vi "Obtain ID from Pool.vi"(8 "error in (no error)":errorcluster, 9 "timeout in ms (0)":i32 format="%d ms", 11 "ID Pool in":refnum<class "ID Pool.lvclass">) -> (0 "error out":errorcluster, 1 "timed out?":bool, 2 "id":i32, 3 "ID Pool out":refnum<class "ID Pool.lvclass">)   [LabVIEW 2017, in "DSF Core.lvlib" / "ID Pool.lvclass"]
uses:
  ID Pool.lvclass
  C:/Git/DSF/Core/Classes/Pool/Pool.lvclass
  Obtain ID Timeout.vi
  Pool.lvclass
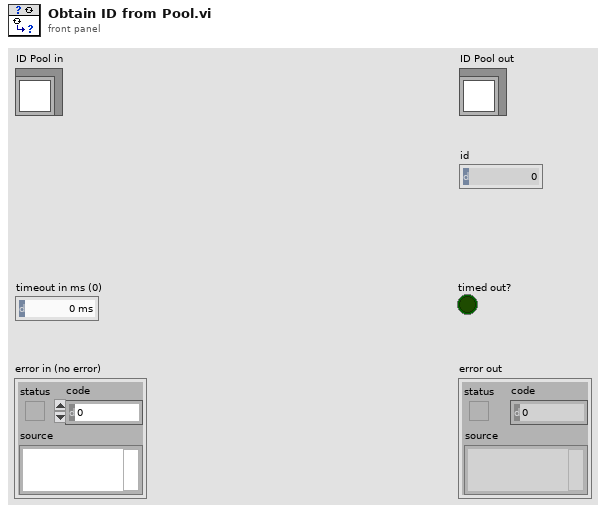
[diagram p1: front panel]
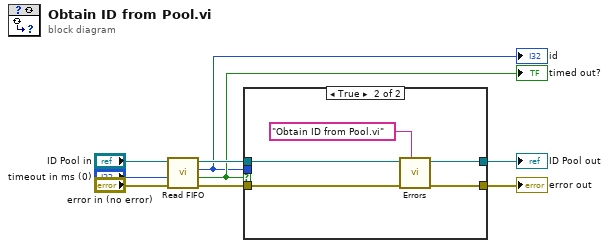
[diagram p0: block diagram]
diagram:
  n1 = call "Read FIFO.vi"("error in (no error)"="error in (no error)", "timeout in ms (0)"="timeout in ms (0)", "Pool in"="ID Pool in") -> ("error out"=w5:errorcluster, "timed out?"=w2:bool, "element"=w1:i32, "Pool out"=w6:refnum<class "ID Pool.lvclass">)  [unwired: 5 in]
  "timed out?" <- w2
  "id" <- w1
  n2 = case shown="True" w2 {
    tunnel: w6 -> [w11 w16]
    tunnel: w5 -> [w10 w15]
    tunnel: [w11 w14] -> w4
    tunnel: [w10 w13] -> w3
    tunnel: w1 -> [_ _]
    frame False {
    }
    frame True {
      n3 = call-poly "Errors.vi"("error source vi name"="Obtain ID from Pool.vi", "error in (no error)"=w15, "ID Pool in"=w16) -> ("error out"=w13:errorcluster, "ID Pool out"=w14:refnum<class "ID Pool.lvclass">)  [unwired: 7 in]
    }
  }
  "error out" <- w3
  "ID Pool out" <- w4
